vi "Fields Populate West Report Fields.vi"(8 "error in (no error)":errorcluster, 11 "Connection Refnum":T1) -> (0 "error out":errorcluster, 2 "Report Field Display Names":T2, 3 "Connection Refnum":T1)   [LabVIEW 2011]
uses:
  DIAdem/Datasheet/Datasheet Field Display Names.ctl
  Summitek EXT/ODBC/SQL Controls/Connection Refnum.ctl
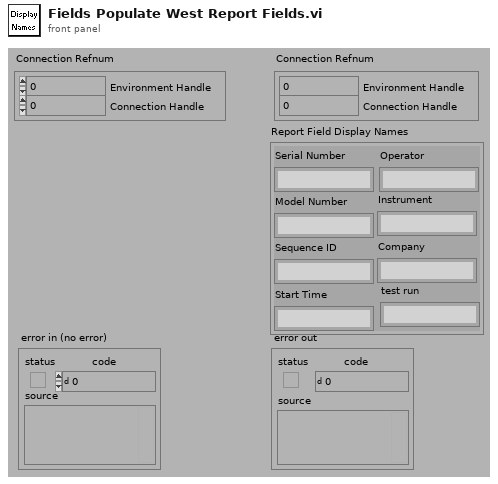
[diagram p1: front panel]
types:
  T1 = typedef "Connection Refnum.ctl" = cluster{"Environment Handle":i32, "Connection Handle":i32}
  T2 = typedef "DATASHEET Field Display Names.ctl" = cluster{"Serial Number":string, "Model Number":string, "Sequence ID":string, "Start Time":string, "Instrument":string, "Company":string, "Operator":string, "test run":string}
  T3 = typedef "Field Record.ctl" = cluster{"ixField":i32, "iSequenceOrder":i32, "sxFieldId":string, "sxSequenceId":string, "sDisplayName":string, "sValue":string, "sUnits":string, "nDataType":T4, "nNextItem":T5, "fSystem":bool, "fSystemValue":bool, "fRequired":bool, "fSetAtTest":bool, "fTestField":bool, "fDeleted":bool, "fIndexed":bool, "fFreeList":bool}
  T4 = typedef "Field DataTypes.ctl" = enum32{"text", "numeric", "list", "timestamp", "boolean"}
  T5 = typedef "Field NextItem.ctl" = enum32{"Reset", "Retain", "Auto-Increment"}
  T6 = cluster{"[0]":string, "[1]":string, "[2]":string, "[3]":string, "[4]":string, "[5]":string, "[6]":string, "[7]":string}
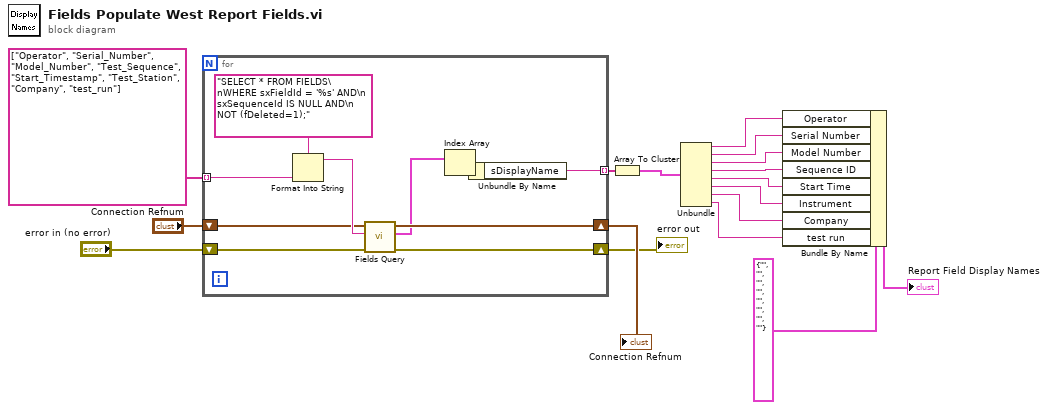
[diagram p0: block diagram]
diagram:
  n1 = for {
    shift-right: [w22] -> w10
    shift-left: "error in (no error)" -> [w26]
    shift-right: [w23] -> w11
    shift-left: "Connection Refnum" -> [w24]
    tunnel: [w19] -> w14 mode=indexing
    tunnel: string[] ["Operator", "Serial_Number", "Model_Number", "Test_Sequence", "Start_Timestamp", "Test_Station", "Company", "test_run"] -> [w18] mode=indexing
    n2 = Format Into String(format string="SELECT * FROM FIELDS\nWHERE sxFieldId = '%s' AND\n  sxSequenceId IS NULL AND\n  NOT (fDeleted=1);" ("Query Name"), w18) -> (resulting string=w25:string)  [unwired: 2 in, 1 out]
    n3 = call "Fields Query.vi"("error in (no error)"=w26, "Query"=w25, "Connection Refnum"=w24) -> ("error out"=w22:errorcluster, "Fields"=w21:T3[], "Connection Refnum"=w23:T1)  [unwired: 1 in, 5 out]
    n4 = Index Array(array=w21) -> (element=w20:T3)  [unwired: 1 in]
    n5 = Unbundle By Name(w20) -> ("sDisplayName"=w19:string)
  }
  "error out" <- w10
  "Connection Refnum" <- w11
  n6 = Array To Cluster(array=w14) -> (cluster=w9:T6)
  n7 = Unbundle(w9) -> ("[0]"=w8:string, "[1]"=w7:string, "[2]"=w6:string, "[3]"=w5:string, "[4]"=w4:string, "[5]"=w3:string, "[6]"=w2:string, "[7]"=w1:string)
  n8 = Bundle By Name(cluster=T2 {"Serial Number"="", "Model Number"="", "Sequence ID"="", "Start Time"="", "Instrument"="", "Company"="", "Operator"="", "test run"=""} ("Report Field Display Names"), "Operator"=w8, "Serial Number"=w7, "Model Number"=w6, "Sequence ID"=w5, "Start Time"=w4, "Instrument"=w3, "Company"=w2, "test run"=w1) -> (→"Report Field Display Names":T2)
